vi "comm set user string.vi"(8 "error in (no error)":errorcluster, 10 "user string":string, 11 "Comm Handle":u32) -> (0 "error out":errorcluster, 3 "dup Comm Handle":u32)   [LabVIEW 2013, in "lvserial.lvlib"]
doc: "Sets user string. The user string is private data value and is unique per serial port. This value is not used by the serial port library for any purpose."
uses:
  lvserial.lvlib
  lvserial.dll
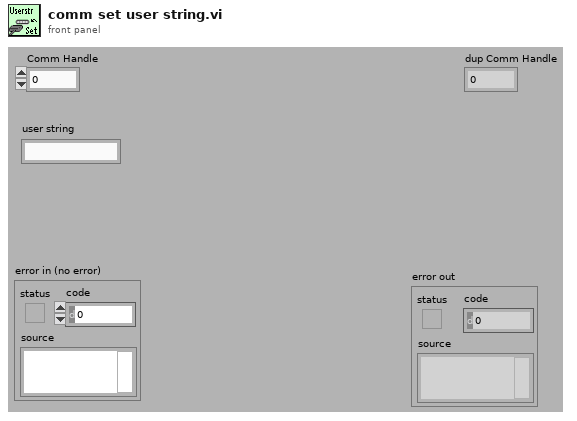
[diagram p1: front panel]
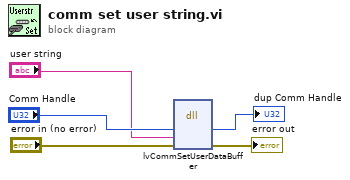
[diagram p0: block diagram]
diagram:
  n1 = dll-call lib="lvserial.dll" fn="lvCommSetUserDataBuffer"("hComm"="Comm Handle", "shUserData"="user string", "error in (no error)"="error in (no error)") -> ("hComm"=→"dup Comm Handle":u32, "error in (no error)"=→"error out":errorcluster)  [unwired: 4 in, 3 out]
